vi "ReadADC_Core.vi"(6 "error in (no error)":errorcluster, 8 "Core PLL Instance":string(combo)="Core0", 9 "ADC to Read":string(combo)="VA") -> (0 "error out":errorcluster, 3 "ADC Value Read":dbl)   [LabVIEW 2011]
doc: "This VI reads a chosen ADC value from the Core PLL instance.\n\nInputs:\n1. ADC to Read: Selects the ADC that will be read through JTAG (ie. LVL, VA, VD, etc.).\n2. Core PLL Instance: Instance of the Core PLL to read the ADC from (Core0, Core1, etc.)\n\nOutputs:\n1.ADC Value Read: The value of the chosen ADC in binary."
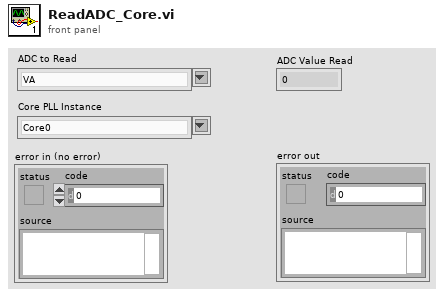
[diagram p1: front panel]
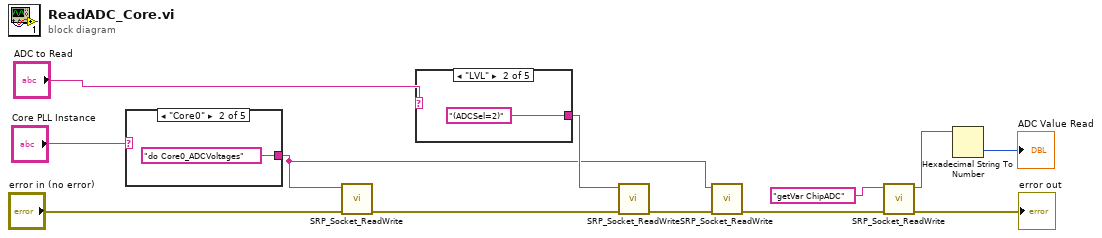
[diagram p0: block diagram]
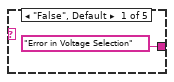
[diagram p2: hidden frame]
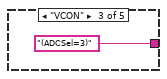
[diagram p3: hidden frame]
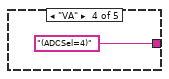
[diagram p4: hidden frame]
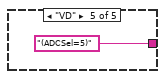
[diagram p5: hidden frame]
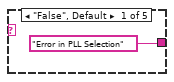
[diagram p6: hidden frame]
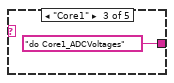
[diagram p7: hidden frame]
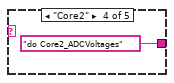
[diagram p8: hidden frame]
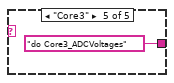
[diagram p9: hidden frame]
diagram:
  n1 = case shown="\"Core0\"" "Core PLL Instance" {
    tunnel: ["Error in PLL Selection" "do Core0_ADCVoltages" "do Core1_ADCVoltages" "do Core2_ADCVoltages" "do Core3_ADCVoltages"] -> w3
    frame "False", Default {
    }
    frame "Core0" {
    }
    frame "Core1" {
    }
    frame "Core2" {
    }
    frame "Core3" {
    }
  }
  n2 = call "SRP_Socket_ReadWrite.vi"("error in (no error)"="error in (no error)", "Data In"=w3) -> ("error out"=w7:errorcluster)  [unwired: 7 in, 1 out]
  n3 = case shown="\"LVL\"" "ADC to Read" {
    tunnel: ["Error in Voltage Selection" "(ADCSel=2)" "(ADCSel=3)" "(ADCSel=4)" "(ADCSel=5)"] -> w4
    frame "False", Default {
    }
    frame "LVL" {
    }
    frame "VCON" {
    }
    frame "VA" {
    }
    frame "VD" {
    }
  }
  n4 = call "SRP_Socket_ReadWrite.vi"("error in (no error)"=w7, "Data In"=w4) -> ("error out"=w8:errorcluster)  [unwired: 7 in, 1 out]
  n5 = call "SRP_Socket_ReadWrite.vi"("error in (no error)"=w8, "Data In"=w3) -> ("error out"=w9:errorcluster)  [unwired: 7 in, 1 out]
  n6 = call "SRP_Socket_ReadWrite.vi"("error in (no error)"=w9, "Data In"="getVar ChipADC") -> ("error out"=→"error out":errorcluster, "Data Out"=w6:string)  [unwired: 7 in]
  n7 = Hexadecimal String To Number(string=w6) -> (number=→"ADC Value Read":u32)  [unwired: 2 in, 1 out]
